vi "Edgertronic-TranslateJSON.vi"(3 "Commands":string[](array[string]), 5 "data":string="HTTP/1.0 200 OK\r\nContent-Type: text/html; charset=utf-8\r\nContent-Length: 313\r\nConnection: close\r\nDate: Tue, 16 Jun 2015 13:54:12 GMT\r\nServer: lighttpd/1.4.11 (edgertonic slow motion camera)\r\n\r\n{\"build_date\": \"20150112\", \"sw_build_date\": \"20140911165611\", \"fpga_initialized\": 1, \"hardware_revision\": 6, \"model_number\": 1, \"home_dir\": \"/home/root/ss-web\", \"ir_filter\": 1, \"mac_addr\": \"00:1B:C5:09:61:4D\", \"serial_console_enabled\": false, \"serial_number\": 333, \"fpga_version\": 70, \"hardware_configuration\": 1}") -> (1 "Values":string[](array[string]))   [LabVIEW 2015]
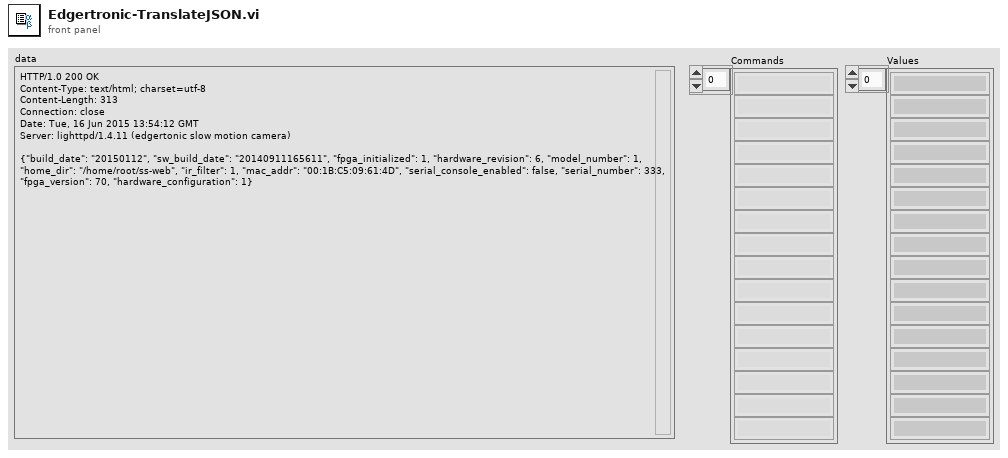
[diagram p1: front panel]
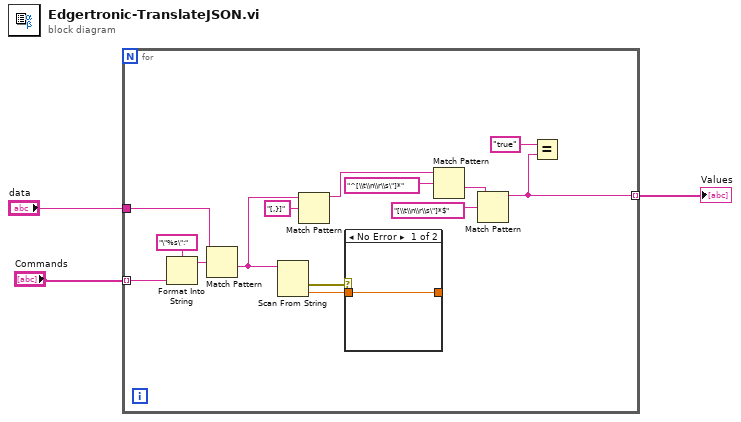
[diagram p0: block diagram]
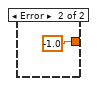
[diagram p2: hidden frame]
diagram:
  n1 = for {
    tunnel: "data" -> [w17]
    tunnel: "Commands" -> [w6] mode=indexing
    tunnel: [w5] -> w2 mode=indexing
    n2 = Format Into String(format string="\"%s\":", w6) -> (resulting string=w15:string)  [unwired: 2 in, 1 out]
    n3 = Match Pattern(string=w17, regular expression=w15) -> (after substring=w4:string)  [unwired: 1 in, 3 out]
    n4 = Scan From String(input string=w4) -> (error out=w12:errorcluster, output 1=w11:dbl)  [unwired: 4 in, 2 out]
    n5 = Match Pattern(string=w4, regular expression="[,}]") -> (before substring=w9:string)  [unwired: 1 in, 3 out]
    n6 = case shown="No Error" w12 {
      tunnel: [w18 -1.0] -> _
      tunnel: w11 -> [w18 _]
      frame No Error {
      }
      frame Error {
      }
    }
    n7 = Match Pattern(string=w9, regular expression="^[\\t\\n\\r\\s\"]*") -> (after substring=w7:string)  [unwired: 1 in, 3 out]
    n8 = Match Pattern(string=w7, regular expression="[\\t\\n\\r\\s\"]*$") -> (before substring=w5:string)  [unwired: 1 in, 3 out]
    n9 = Equal?(x="true", y=w5) -> ()  [unwired: 1 out]
  }
  "Values" <- w2
